vi "zapiszWspolrzednePionowe.vi"(9 "Lista punktów w pionie":i32[](array[numeric]), 10 "K¹t uœredniony":i32, 11 "Wybór komory":T1) -> ()   [LabVIEW 2014]
uses:
  parametryKomorVIs/WyborKomory.ctl
  AkcjaGFV.ctl
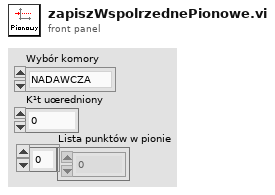
[diagram p1: front panel]
types:
  T1 = typedef "WyborKomory.ctl" = enum16{"NADAWCZA", "ODBIORCZA"}
  T2 = typedef "AkcjaGFV.ctl" = enum16{"Czytaj", "Zapisz", "Reset"}
  T3 = typedef "WyjsciaParametry.ctl" = cluster{"Nad. lewo":bool, "Nad.  prawo":bool, "Nad.  gora":bool, "Nad. do³":bool, "Dzialanie":bool, "Pomiar":bool, "Odb. lewo":bool, "Odb.  prawo":bool, "Odb.  gora":bool, "Odb. dol":bool, "Pozostalo punktow":i32, "Nad. elewacja":i32, "Nad. azymut":i32, "Odb. elewacja":i32, "Odb. azymut":i32, "TCP Error":bool, "TCP Error Code":i32, "LINX Error":bool, "LINX Error Code":i32, "Nastepny elewacja":i32, "Nastepny azymut":i32, "Coords Error":bool, "Inicjalizacja pozycji":bool}
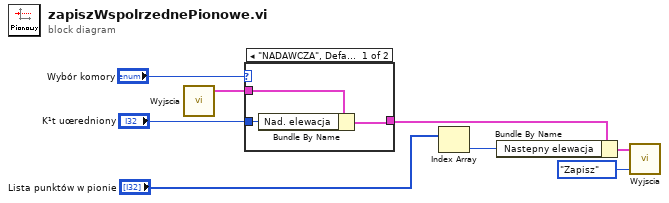
[diagram p0: block diagram]
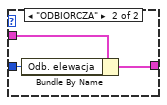
[diagram p2: hidden frame]
diagram:
  n1 = call "Wyjscia.vi"() -> ("Wyjœcie"=w8:T3)  [unwired: 5 in]
  n2 = case shown="\"NADAWCZA\", Default" "Wybór komory" {
    tunnel: w8 -> [w11 w13]
    tunnel: "K¹t uœredniony" -> [w10 w12]
    tunnel: [w9 w14] -> w1
    frame "NADAWCZA", Default {
      n3 = Bundle By Name(cluster=w11, "Nad. elewacja"=w10) -> (w9:T3)
    }
    frame "ODBIORCZA" {
      n4 = Bundle By Name(cluster=w13, "Odb. elewacja"=w12) -> (w14:T3)
    }
  }
  n5 = Index Array(array="Lista punktów w pionie") -> (element=w7:i32)  [unwired: 1 in]
  n6 = Bundle By Name(cluster=w1, "Nastepny elewacja"=w7) -> (w6:T3)
  n7 = call "Wyjscia.vi"("Akcja"=AkcjaGFV."Zapisz", "Wejœcie"=w6) -> ()  [unwired: 3 in, 1 out]
